vi "Arm and Set Trigger - Transient.vi"(8 "error in":errorcluster, 11 "Carrier Connection In":T1={"Description"="", "Address"="", "Port"=0, "timeout (ms)"=5000, "Termination Character"="\n", "TCP Connection Reference"=refnum, "Open Connection"=FALSE}) -> (0 "error out":errorcluster, 3 "DTACQ Connection Out":T1)   [LabVIEW 2017, in "DTACQ - Network Enabled Device Driver.lvlib"]
doc: "Arms and fires a transient shot. Waits until data is ready for downoad, before exiting the VI."
uses:
  DTACQ - Network Enabled Device Driver.lvlib
  Communications/Typedefs/DTACQ Connection Data--Cluster.ctl
  Communications/Communications Library.lvlib
panel:
  in  "ARM":bool
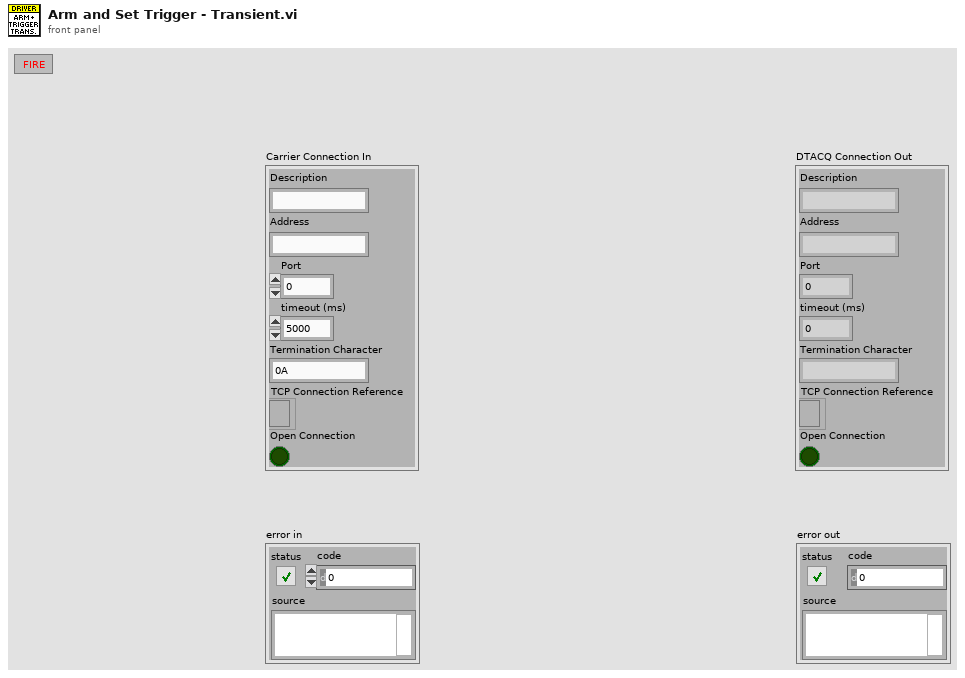
[diagram p1: front panel]
types:
  T1 = typedef "Communications Library.lvlib/DTACQ Connection Data--Cluster.ctl" = cluster{"Description":string, "Address":string, "Port":u16, "timeout (ms)":i32, "Termination Character":string, "TCP Connection Reference":refnum<k5>, "Open Connection":bool}
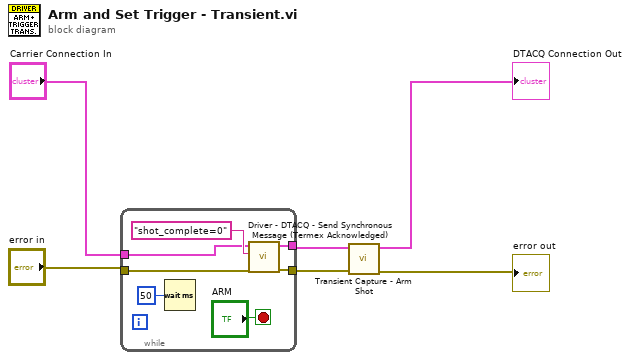
[diagram p0: block diagram]
diagram:
  n1 = while {
    tunnel: "error in" -> [w11]
    tunnel: [w10] -> w5
    tunnel: "Carrier Connection In" -> [w9]
    tunnel: [w8] -> w2
    stop <- "ARM" stop-if-true
    n2 = Wait (ms)(milliseconds to wait=u32 50) -> ()  [unwired: 1 out]
    n3 = call "Driver - DTACQ - Send Synchronous Message (Termex Acknowledged).vi"("error in"=w11, "Message to Send"="shot_complete=0", "DTACQ Connection Data In"=w9) -> ("error out"=w10:errorcluster, "DTACQ Connection Data Out"=w8:T1)  [unwired: 5 in, 2 out]
  }
  n4 = call "Transient Capture - Arm Shot.vi"("error in"=w5, "Carrier Connection Out"=w2) -> ("error out"=→"error out":errorcluster, "DTACQ Connection Out"=→"DTACQ Connection Out":T1)  [unwired: 8 in]
